vi "ESC_CmdStr.vi"(1 "ESC状态":T1 {"AVH提示状态" items=["关", "介入", "待机", "错误"]; "ABS_ESC信号提示车速" min=0.0 max=491.34 step=0.06 scale=0.0..491.34 scale format="%#_8f"}) -> (0 "CmdStr":string)   [LabVIEW 2013]
uses:
  ESC_125.ctl
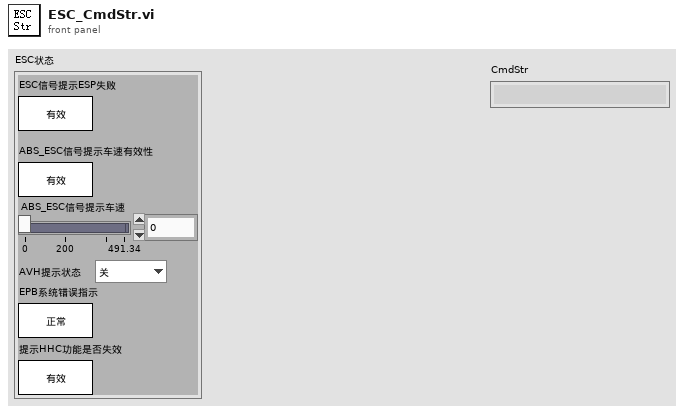
[diagram p1: front panel]
types:
  T1 = typedef "ESC_125.ctl" = cluster{"ESC信号提示ESP失败":bool, "ABS_ESC信号提示车速有效性":bool, "ABS_ESC信号提示车速":dbl, "AVH提示状态":u16, "EPB系统错误指示":bool, "提示HHC功能是否失效":bool}
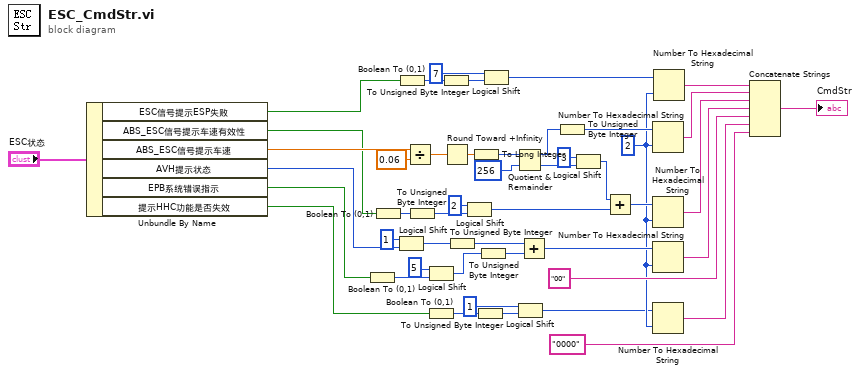
[diagram p0: block diagram]
diagram:
  w5 = 2
  n1 = Unbundle By Name("ESC状态") -> ("ESC信号提示ESP失败"=w28:bool, "ABS_ESC信号提示车速有效性"=w29:bool, "ABS_ESC信号提示车速"=w30:dbl, "AVH提示状态"=w22:u16, "EPB系统错误指示"=w20:bool, "提示HHC功能是否失效"=w6:bool)
  n2 = Boolean To (0,1)(Boolean=w20) -> (0, 1=w16:i16)
  n3 = Boolean To (0,1)(Boolean=w29) -> (0, 1=w40:i16)
  n4 = Logical Shift(y=u8 1, x=w22) -> (x << y=w21:u16)
  n5 = Boolean To (0,1)(Boolean=w28) -> (0, 1=w27:i16)
  n6 = Divide(x=w30, y=0.06) -> (x/y=w46:dbl)
  n7 = To Unsigned Byte Integer(number=w40) -> (unsigned 8bit integer=w13:u8)
  n8 = Logical Shift(y=u8 5, x=w16) -> (x << y=w17:i16)
  n9 = Boolean To (0,1)(Boolean=w6) -> (0, 1=w7:i16)
  n10 = To Unsigned Byte Integer(number=w27) -> (unsigned 8bit integer=w14:u8)
  n11 = Round Toward +Infinity(x=w46) -> (ceil(x): smallest int >= x=w44:dbl)
  n12 = To Unsigned Byte Integer(number=w21) -> (unsigned 8bit integer=w12:u8)
  n13 = Logical Shift(y=u8 2, x=w13) -> (x << y=w36:u8)
  n14 = To Long Integer(number=w44) -> (32bit integer=w43:i32)
  n15 = To Unsigned Byte Integer(number=w7) -> (unsigned 8bit integer=w9:u8)
  n16 = To Unsigned Byte Integer(number=w17) -> (unsigned 8bit integer=w11:u8)
  n17 = Logical Shift(y=u8 7, x=w14) -> (x << y=w25:u8)
  n18 = Quotient & Remainder(x=w43, y=256) -> (x-y*floor(x/y)=w38:i32, floor(x/y)=w39:i32)
  n19 = Logical Shift(y=u8 1, x=w9) -> (x << y=w4:u8)
  n20 = Add(x=w12, y=w11) -> (x+y=w19:u8)
  n21 = To Unsigned Byte Integer(number=w38) -> (unsigned 8bit integer=w35:u8)
  n22 = Logical Shift(y=i16 3, x=w39) -> (x << y=w37:i32)
  n23 = Add(x=w37, y=w36) -> (x+y=w34:i32)
  n24 = Number To Hexadecimal String(1:w5, 2:w35) -> (0:w33:string)
  n25 = Number To Hexadecimal String(1:w5, 2:w34) -> (0:w32:string)
  n26 = Number To Hexadecimal String(1:w5, 2:w19) -> (0:w18:string)
  n27 = Number To Hexadecimal String(1:w5, 2:w4) -> (0:w3:string)
  n28 = Number To Hexadecimal String(1:w5, 2:w25) -> (0:w24:string)
  n29 = Concatenate Strings(w24, w33, w32, w18, "00", w3, "0000") -> (→"CmdStr":string)
